vi "Teleop.vi"(10 "Match Info":T1={"Autonomous Elapsed Seconds"=0.0, "TeleOp Elapsed Seconds"=0.0, "Disabled Elapsed Seconds"=0.0, "Visited Autonomous"=FALSE, "Visited TeleOp"=FALSE, "Visited Disabled"=FALSE, "Autonomous Settings"={"Autonomous Style"=enum."Independent", "VI Refnum"=refnum}}, 11 "Call Context":T2) -> ()   [LabVIEW 2016]
doc: "This VI is called for each TeleOp packet received from the DS where the robot is not disabled. It is often used to read from the joysticks and update I/O or to update setpoints for timed control loops. It should complete and return within 20 milliseconds or it may miss DS packets."
uses:
  Controllers.ctl
  Robot Global Data.vi
  <vilib>/Rock Robotics/WPI/DriverStation/WPI_DriverStationDerivedRobotMode.ctl
  <vilib>/Rock Robotics/WPI/DriverStation/WPI_DriverStationMatch Info.ctl
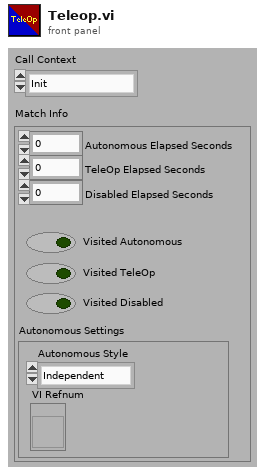
[diagram p1: front panel]
types:
  T1 = typedef "WPI_DriverStationMatch Info.ctl" = cluster{"Autonomous Elapsed Seconds":dbl, "TeleOp Elapsed Seconds":dbl, "Disabled Elapsed Seconds":dbl, "Visited Autonomous":bool, "Visited TeleOp":bool, "Visited Disabled":bool, "Autonomous Settings":cluster{"Autonomous Style":enum16{"Iterative", "Independent"}, "VI Refnum":refnum<vi>}}
  T2 = typedef "WPI_DriverStationDerivedRobotMode.ctl" = enum16{"Init", "Execute", "Stop"}
  T3 = cluster{"X":dbl, "Y":dbl, "Z":dbl, "B (straight drive)":bool, "T1 Climber Up":bool}
  T4 = typedef "Controllers.ctl" = enum16{"Controller", "Controller2"}
  T5 = typedef "WPI_JoystickDevRef.ctl" = cluster{"Device":T6}
  T6 = typedef "WPI_JoystickDeviceEnum.ctl" = enum16{"USB 0", "USB 1", "USB 2", "USB 3", "USB 4", "USB 5"}
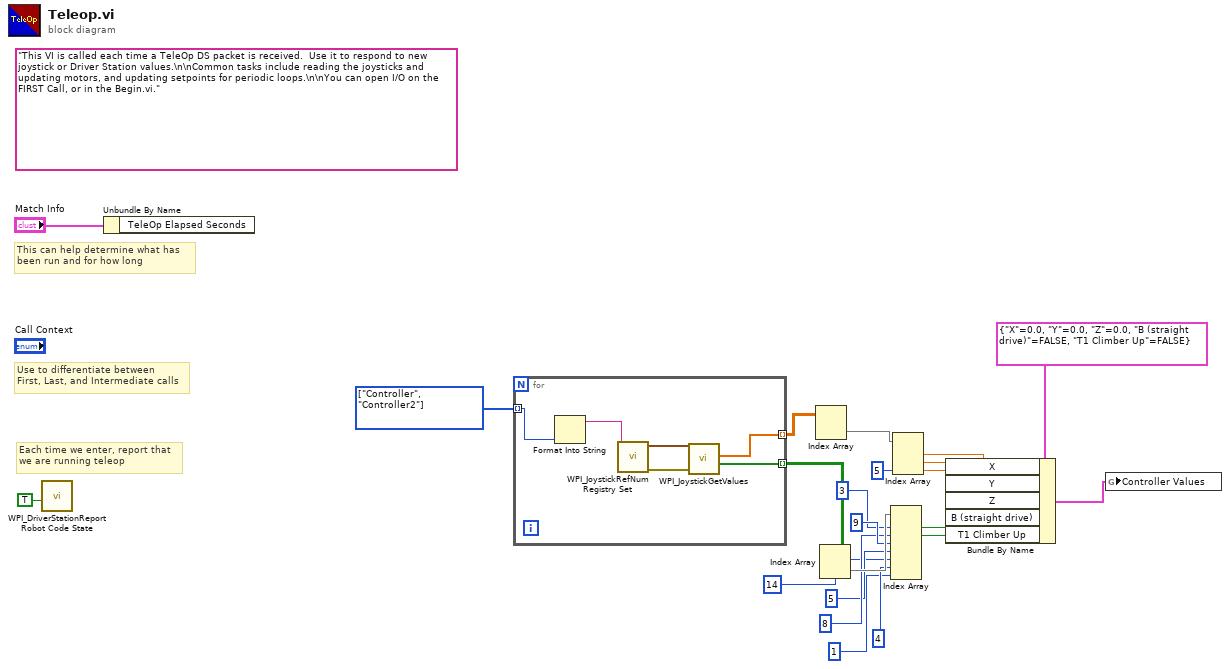
[diagram p0: block diagram]
diagram:
  w20 = T4[] [enum."Controller", enum."Controller2"] items=["Controller", "Controller2"]
  (unwired) "This VI is called each time a TeleOp DS packet is received.  Use it to respond to new joystick or Driver Station values.\n\nCommon tasks include reading the joysticks and updating motors, and updating setpoints for periodic loops.\n\nYou can open I/O on the FIRST Call, or in the Begin.vi."
  # "Each time we enter, report that\nwe are running teleop"
  # "Use to differentiate between\nFirst, Last, and Intermediate calls"
  # "This can help determine what has\nbeen run and for how long"
  n1 = call <vilib>:"WPI_DriverStationReport Robot Code State.vi"("TeleOp"=TRUE ("Autonomous")) -> ()  [unwired: 10 in, 1 out]
  n2 = Unbundle By Name("Match Info") -> ()  [unwired: 1 out]
  n3 = for {
    tunnel: w20 -> [w28] mode=indexing
    tunnel: [w24] -> w14 mode=indexing
    tunnel: [w23] -> w19 mode=indexing
    n4 = Format Into String(w28) -> (resulting string=w25:string)  [unwired: 3 in, 1 out]
    n5 = call <vilib>:"WPI_JoystickRefNum Registry Set.vi"("refnum name"=w25) -> ("error out"=w26:errorcluster, "JoystickDevRef"=w27:T5)  [unwired: 9 in]
    n6 = call <vilib>:"WPI_JoystickGetValues.vi"("error in (no error)"=w26, "JoystickDevRef"=w27) -> ("Buttons"=w24:bool[], "Axes"=w23:dbl[])  [unwired: 5 in, 3 out]
  }
  n7 = Index Array(array=w19) -> (element=w18:dbl[])  [unwired: 2 in]
  n8 = Index Array(array=w14) -> (element=w13:bool[])  [unwired: 2 in]
  n9 = Index Array(array=w13, index #1=3 ("index"), index #2=8 ("index"), index #3=9 ("index"), index #4=5 ("index"), index #5=14 ("index"), index #6=4 ("index"), index #7=1 ("index")) -> (element #1=w2:bool, element #2=w1:bool)  [unwired: 5 out]
  n10 = Index Array(array=w18, index #3=5 ("index")) -> (element #1=w12:dbl, element #2=w11:dbl, element #3=w10:dbl)  [unwired: 2 in]
  n11 = Bundle By Name(cluster=T3 {"X"=0.0, "Y"=0.0, "Z"=0.0, "B (straight drive)"=FALSE, "T1 Climber Up"=FALSE} ("input cluster"), "X"=w12, "Y"=w11, "Z"=w10, "B (straight drive)"=w2, "T1 Climber Up"=w1) -> (w15:T3)
  n12 = global write "Robot Global Data.vi" "Controller Values"(w15) -> ()
